vi "Test Sweep Manager Subsystems.vi"(8 "error in (no error)":errorcluster, 11 "Generator in":refnum<class "Generator.lvclass">) -> (0 "error out":errorcluster, 3 "Generator out":refnum<class "Generator.lvclass">)   [LabVIEW 2019, in "Generator.lvclass"]
uses:
  Generator.lvclass
  typedefs/AO.Channel--Cluster--Array.ctl
  typedefs/AO.Channel--Cluster.ctl
  typedefs/AO.Channel.Function--Enum.ctl
  typedefs/Sampling--Cluster.ctl
  typedefs/Sweep.Configuration--Cluster.ctl
  typedefs/Sweep.Channel--Cluster--Array.ctl
  typedefs/Sweep.Channel--Cluster.ctl
  typedefs/Sweep.Pattern--Enum.ctl
  Generator.lvclass/Generator.ctl
panel:
  out "Sweep Graph":waveform(dbl)[](graph)
  in  "Sweep Tables":cluster{"Channel":u16, "Sweep Pattern":dbl[]}[](array[cluster])=[{"Channel"=4, "Sweep Pattern"=[0.01, 0.02, 0.015, 0.025, 0.02, 0.03]}] {"Sweep Pattern" format="%#_3p"; "Channel" min=1 max=128}
  in  "milliseconds to wait":u32=100
  out "Updates":i32=13
  out "Update #":i32=12
  out "Waveform Graph":waveform(dbl)[](graph)
  in  "Configuration.Sweep":T1={"Sweep Time (s)"=100.0, "Initial Wait (s)"=0.1, "Return to Start"=TRUE, "Channels"=[{"Enable?"=TRUE, "Channel"=1, "Start"=0.0, "End"=0.1, "Pattern"=enum."Smooth Ramp _/\\_", "Table"=[]}, {"Enable?"=TRUE, "Channel"=2, "Start"=0.09, "End"=0.09, "Pattern"=enum."Smooth Ramp _/\\_", "Table"=[]}, {"Enable?"=TRUE, "Channel"=3, "Start"=0.0, "End"=0.01, "Pattern"=enum."Ramp /\\", "Table"=[]}, {"Enable?"=TRUE, "Channel"=4, "Start"=0.01, "End"=0.011, "Pattern"=enum."Table", "Table"=[]}]} {"Channels"."Table" format="%#_1f"; "Channels"."Channel" min=1 max=128; "Channels"."Start" format="%#_6p"; "Channels"."End" format="%#_6p"}
  in  "Sampling":T5={"Fs"=10000.0, "#s"=1000.0}
  in  "stop":bool
  in  "AO Channels":T6=[{"Enable?"=TRUE, "Channel"=1, "Amplitude"=0.1, "Offset"=0.0, "Frequency"=13.0, "Phase"=0.0, "Function"=enum."sine", "Sweeping?"=FALSE, "Limit AC?"=FALSE, "Limit DC?"=FALSE, "Duty Cycle?"=FALSE, "Duty Cycle"=0.0}, {"Enable?"=TRUE, "Channel"=0, "Amplitude"=0.0, "Offset"=0.09, "Frequency"=0.1, "Phase"=0.0, "Function"=enum."sine", "Sweeping?"=FALSE, "Limit AC?"=FALSE, "Limit DC?"=FALSE, "Duty Cycle?"=FALSE, "Duty Cycle"=0.0}, {"Enable?"=TRUE, "Channel"=0, "Amplitude"=0.0, "Offset"=0.0, "Frequency"=0.1, "Phase"=0.0, "Function"=enum."sine", "Sweeping?"=FALSE, "Limit AC?"=FALSE, "Limit DC?"=FALSE, "Duty Cycle?"=FALSE, "Duty Cycle"=0.0}, {"Enable?"=TRUE, "Channel"=0, "Amplitude"=0.0, "Offset"=0.01, "Frequency"=0.1, "Phase"=0.0, "Function"=enum."sine", "Sweeping?"=FALSE, "Limit AC?"=FALSE, "Limit DC?"=FALSE, "Duty Cycle?"=FALSE, "Duty Cycle"=0.0}]
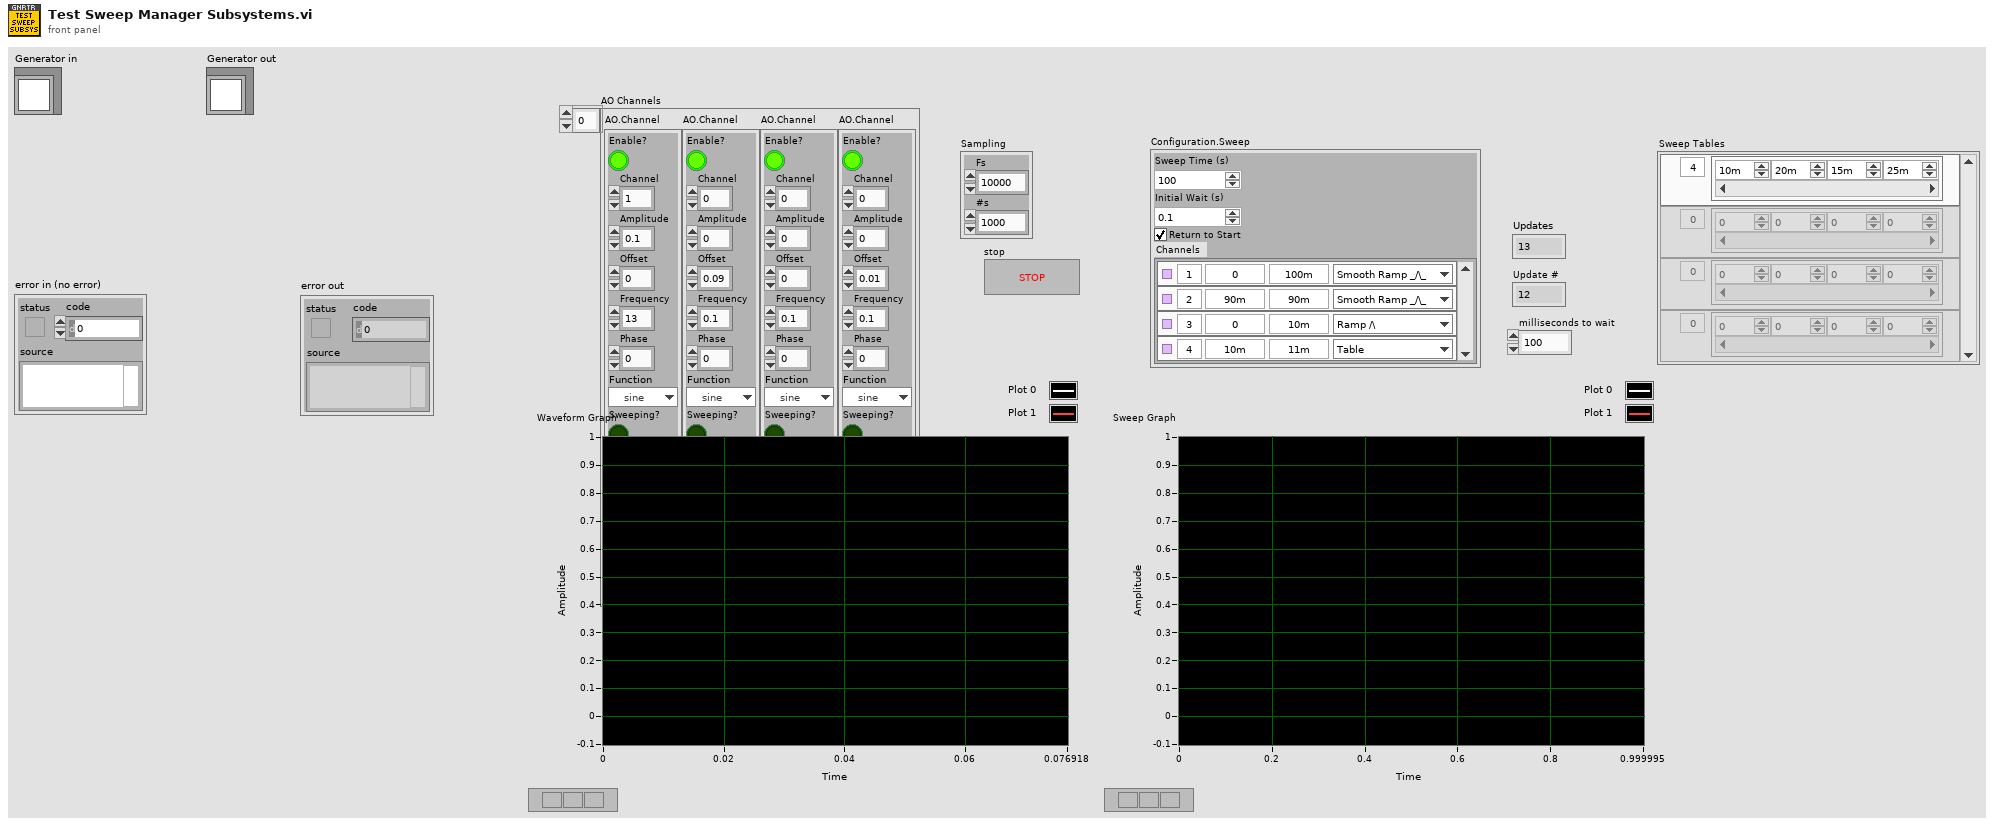
[diagram p1: front panel]
types:
  T1 = typedef "Generator.lvclass/Sweep.Configuration--Cluster.ctl" = cluster{"Sweep Time (s)":dbl, "Initial Wait (s)":dbl, "Return to Start":bool, "Channels":T2}
  T2 = typedef "Generator.lvclass/Sweep.Channel--Cluster--Array.ctl" = T3[]
  T3 = typedef "Generator.lvclass/Sweep.Channel--Cluster.ctl" = cluster{"Enable?":bool, "Channel":u16, "Start":dbl, "End":dbl, "Pattern":T4, "Table":dbl[]}
  T4 = typedef "Generator.lvclass/Sweep.Pattern--Enum.ctl" = enum16{"Ramp /", "Ramp /\\", "Smooth Ramp _/", "Smooth Ramp _/\\_", "Table"}
  T5 = typedef "Generator.lvclass/Sampling--Cluster.ctl" = cluster{"Fs":dbl, "#s":dbl}
  T6 = typedef "Generator.lvclass/AO.Channel--Cluster--Array.ctl" = T7[]
  T7 = typedef "Generator.lvclass/AO.Channel--Cluster.ctl" = cluster{"Enable?":bool, "Channel":i32, "Amplitude":dbl, "Offset":dbl, "Frequency":dbl, "Phase":dbl, "Function":T8, "Sweeping?":bool, "Limit AC?":bool, "Limit DC?":bool, "Duty Cycle?":bool, "Duty Cycle":dbl}
  T8 = typedef "Generator.lvclass/AO.Channel.Function--Enum.ctl" = enum16{"sine", "square", "triangle", "saw"}
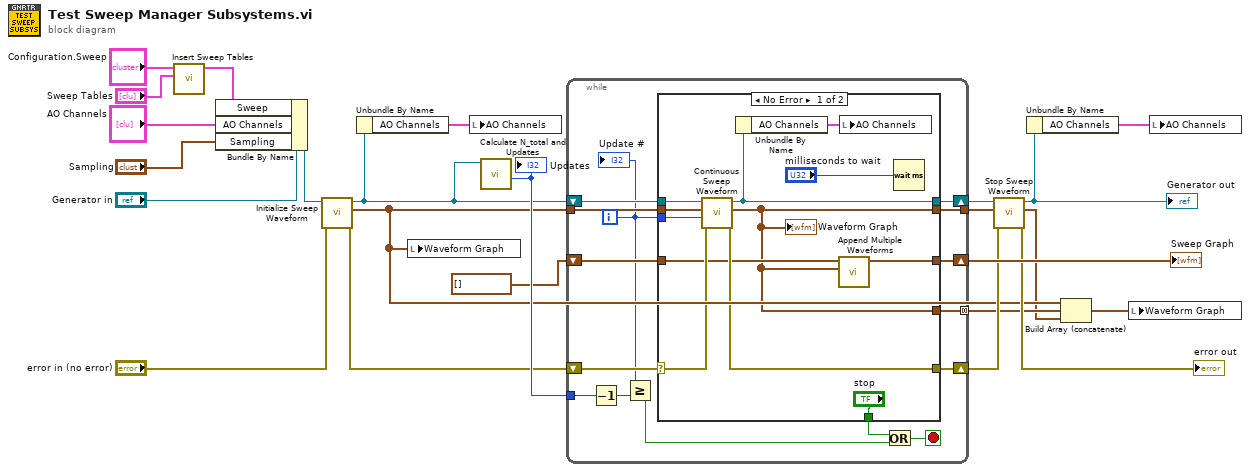
[diagram p0: block diagram]
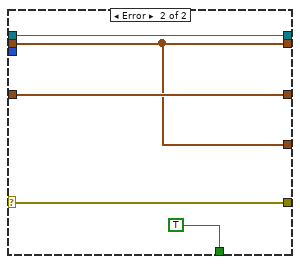
[diagram p2: hidden frame]
diagram:
  n1 = call "Insert Sweep Tables.vi"("Channels New"="Sweep Tables", "Sweep Configuration in"="Configuration.Sweep") -> ("Sweep Configuration out"=w17:T1)  [unwired: 9 in]
  n2 = Bundle By Name(cluster="Generator in", "Sweep"=w17, "AO Channels"="AO Channels", "Sampling"="Sampling") -> (w20:refnum<class "Generator.lvclass">)
  n3 = call "Initialize Sweep Waveform.vi"("error in (no error)"="error in (no error)", "Generator in"=w20) -> ("error out"=w11:errorcluster, "Waveforms"=w3:waveform(dbl)[], "Generator out"=w15:refnum<class "Generator.lvclass">)  [unwired: 7 in]
  n4 = Unbundle By Name(w15) -> ("AO Channels"=w14:T6)
  n5 = local write "Waveform Graph"(w3) -> ()
  n6 = local write "AO Channels"(w14) -> ()
  n7 = call "Calculate N_total and Updates.vi"("Generator in"=w15) -> ("Updates"=w19:i32)  [unwired: 8 in, 2 out]
  "Updates" <- w19
  n8 = while {
    shift-right: [w38] -> w7
    shift-left: w11 -> [w39]
    shift-right: [w36] -> w9
    shift-left: w15 -> [w37]
    tunnel: w3 -> [w35]
    tunnel: w19 -> [w34]
    shift-right: [w29] -> w12
    shift-left: waveform(dbl)[] [] ("Waveform out []") -> [w28]
    tunnel: [w26] -> w5
    tunnel: [w25] -> w4 mode=concatenating
    i -> [w27]
    stop <- w31 stop-if-true
    n9 = Decrement(x=w34) -> (x-1=w30:i32)
    n10 = Greater Or Equal?(x=w27, y=w30) -> (x >= y?=w33:bool)
    n11 = case shown="No Error" w39 {
      selector: w39 -> [w47 w56]
      tunnel: [w50 w56] -> w38
      tunnel: [w43 w55] -> w36
      tunnel: w37 -> [w48 w55]
      tunnel: ["stop" TRUE ("stop")] -> w32
      tunnel: w35 -> [w49 w52]
      tunnel: w27 -> [w46 _]
      tunnel: [w41 w53] -> w29
      tunnel: w28 -> [w42 w53]
      tunnel: [w40 w52] -> w26
      tunnel: [w40 w52] -> w25
      frame No Error {
        n12 = call "Continuous Sweep Waveform.vi"("error in (no error)"=w47, "Sweep Index"=w46, "Waveforms in"=w49, "Generator in"=w48) -> ("error out"=w50:errorcluster, "Waveforms out"=w40:waveform(dbl)[], "Generator in"=w43:refnum<class "Generator.lvclass">)  [unwired: 4 in, 1 out]
        "Waveform Graph" <- w40
        n13 = Unbundle By Name(w43) -> ("AO Channels"=w44:T6)
        n14 = call "Append Multiple Waveforms.vi"("Waveform B []"=w40, "Waveforrm A []"=w42) -> ("Waveform out []"=w41:waveform(dbl)[])  [unwired: 8 in, 1 out]
        n15 = local write "AO Channels"(w44) -> ()
        n16 = Wait (ms)(milliseconds to wait="milliseconds to wait") -> ()  [unwired: 1 out]
      }
      frame Error {
      }
    }
    n17 = Or(x=w32, y=w33) -> (x .or. y?=w31:bool)
    "Update #" <- w27
  }
  "Sweep Graph" <- w12
  n18 = call "Stop Sweep Waveform.vi"("error in (no error)"=w7, "Waveforms in"=w5, "Generator in"=w9) -> ("error out"=→"error out":errorcluster, "Waveforms out"=w2:waveform(dbl)[], "Generator out"=w8:refnum<class "Generator.lvclass">)  [unwired: 6 in]
  "Generator out" <- w8
  n19 = Unbundle By Name(w8) -> ("AO Channels"=w13:T6)
  n20 = Build Array (concatenate)(w3, w4, w2) -> (w1:waveform(dbl)[])
  n21 = local write "Waveform Graph"(w1) -> ()
  n22 = local write "AO Channels"(w13) -> ()
